vi "GetInstrumentVIs.vi"(8 "error in (no error)":errorcluster, 10 "InstrContaining":path[](array[path]), 11 "DestinationDirectory":path) -> (0 "error out":errorcluster, 3 "InstrContainingVI[]":path[](array[path]))   [LabVIEW 2021, in "Converter.lvlib"]
uses:
  Converter.lvlib
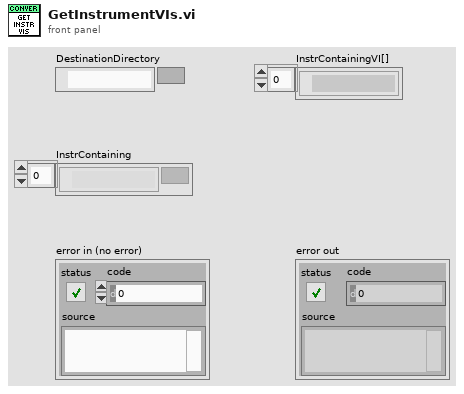
[diagram p1: front panel]
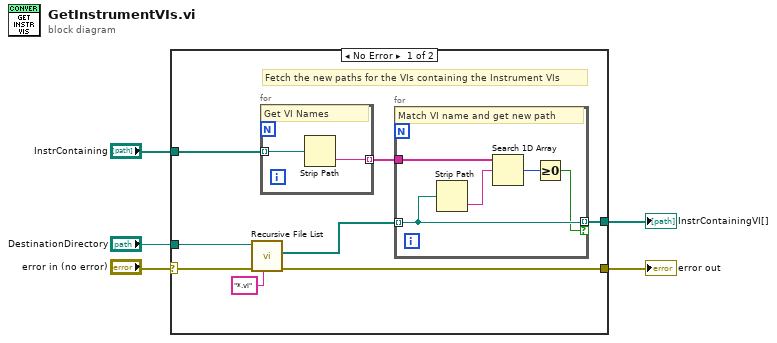
[diagram p0: block diagram]
diagram:
  n1 = case shown="No Error" "error in (no error)" {
    selector: "error in (no error)" -> [w8 w21]
    tunnel: [w13 w21] -> w5
    tunnel: [w12 _] -> w4
    tunnel: "InstrContaining" -> [w11 _]
    tunnel: "DestinationDirectory" -> [w7 _]
    frame No Error {
      # "Fetch the new paths for the VIs containing the Instrument VIs"
      n2 = call <vilib>:"Recursive File List.vi"("pattern"="*.vi", "error in (no error)"=w8, "Folder Path"=w7) -> ("error out"=w13:errorcluster, "All Files in Dir"=w9:path[])  [unwired: 4 in, 3 out]
      n3 = for {
        tunnel: w11 -> [w15] mode=indexing
        tunnel: [w14] -> w10 mode=indexing
        # "Get VI Names"
        n4 = Strip Path(path=w15) -> (name=w14:string)  [unwired: 1 out]
      }
      n5 = for {
        tunnel: w9 -> [w17] mode=indexing
        tunnel: w10 -> [w20]
        tunnel: [w17] -> w12 mode=indexing if=w16
        # "Match VI name and get new path"
        n6 = Strip Path(path=w17) -> (name=w19:string)  [unwired: 1 out]
        n7 = Search 1D Array(1D array=w20, element=w19) -> (index of element=w18:i32)  [unwired: 1 in]
        n8 = Greater Or Equal To 0?(x=w18) -> (x >= 0?=w16:bool)
      }
    }
    frame Error {
    }
  }
  "error out" <- w5
  "InstrContainingVI[]" <- w4
